vi "Get Front Panel Reference.vi"(8 "error in (no error)":errorcluster, 11 "MenuButton Event Handler in":refnum<class "MenuButton Event Handler.lvclass">) -> (0 "error out":errorcluster, 3 "MenuButton Event Handler out":refnum<class "MenuButton Event Handler.lvclass">)   [LabVIEW 2017, in "MenuButtons.lvlib" / "MenuButton Event Handler.lvclass"]
uses:
  MenuButton Event Handler.lvclass
  MenuButton Event Handler.lvclass/MenuButton Event Handler.ctl
  MenuButton/MenuButton.lvclass/MenuButton.ctl
  MenuButton/MenuButton.lvclass
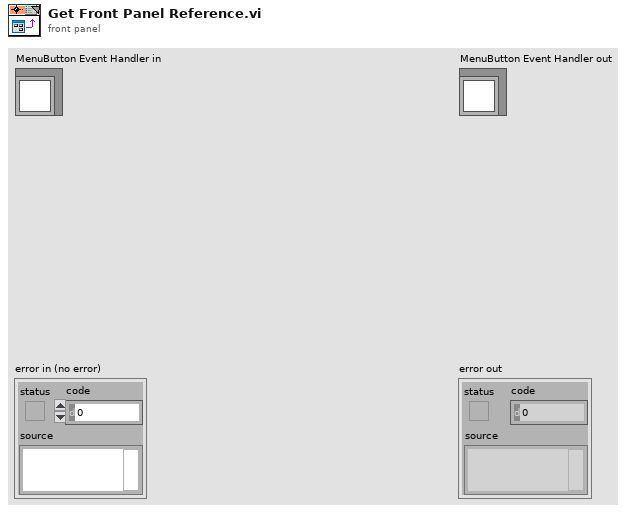
[diagram p1: front panel]
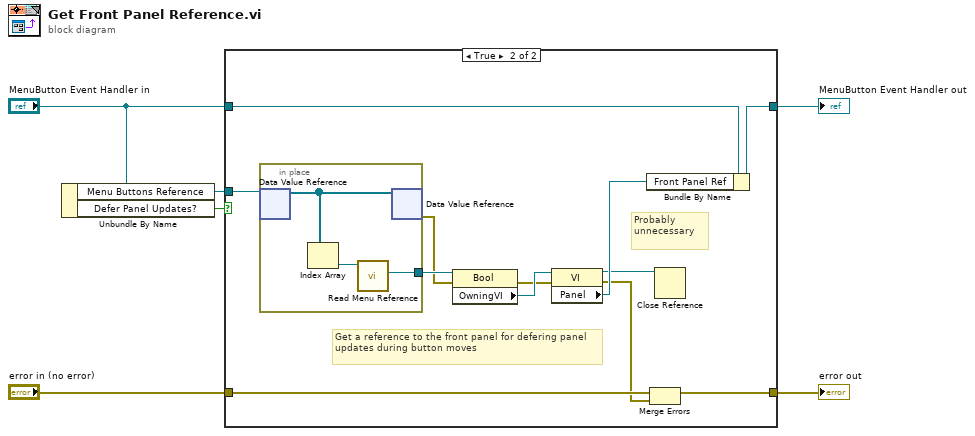
[diagram p0: block diagram]
diagram:
  n1 = Unbundle By Name("MenuButton Event Handler in") -> ("Menu Buttons Reference"=w6:refnum<data-value>, "Defer Panel Updates?"=w5:bool)
  n2 = case shown="True" w5 {
    tunnel: w6 -> [_ w20]
    tunnel: "MenuButton Event Handler in" -> [w8 w19]
    tunnel: [w8 w17] -> w3
    tunnel: "error in (no error)" -> [w7 w12]
    tunnel: [w7 w11] -> w1
    frame False {
      # "Not configured to defer panel updates - I made this optional to allow flexibility - the caller may want to explicitly defer and resume panel updates based actions beyond the scope of this class."
    }
    frame True {
      # "Get a reference to the front panel for defering panel updates during button moves"
      # "Probably unnecessary"
      n3 = in-place {
        in-place-border: [w21] -> w18
        n4 = in-place-dvr #1(w20) -> (w23:refnum<class "MenuButton.lvclass">[])  [unwired: 1 out]
        n5 = Index Array(array=w23) -> (element=w22:refnum<class "MenuButton.lvclass">)  [unwired: 1 in]
        n6 = call "Read Menu Reference.vi"("MenuButton in"=w22) -> ("Menu Reference"=w21:refnum<vi>)  [unwired: 8 in, 2 out]
        n7 = in-place-dvr #1(w23) -> (w15:errorcluster)  [unwired: 1 out]
      }
      n8 = property class="Bool"(reference=w18, error in=w15) -> (error out=w14:errorcluster, "OwningVI"=w16:refnum<vi>)  [unwired: 1 out]
      n9 = property class="VI"(reference=w16, error in=w14) -> (reference out=w9:refnum<vi>, error out=w10:errorcluster, "Panel"=w13:refnum<vi>)
      n10 = Bundle By Name(cluster=w19, "Front Panel Ref"=w13) -> (w17:refnum<class "MenuButton Event Handler.lvclass">)
      n11 = Merge Errors(w12, w10) -> (w11:errorcluster)
      n12 = Close Reference(reference=w9) -> ()  [unwired: 1 in, 1 out]
    }
  }
  "error out" <- w1
  "MenuButton Event Handler out" <- w3
